vi "Momentum_Killer_V2.vi"(4 "Reverse Power":dbl, 5 "Stop Delay (sec)":dbl=0.5, 6 "Reverse Time (sec)":dbl, 7 "Edge":bool, 9 "Kill Control":bool, 11 "Power Input":dbl) -> (3 "Power Output":dbl)   [LabVIEW 2016]
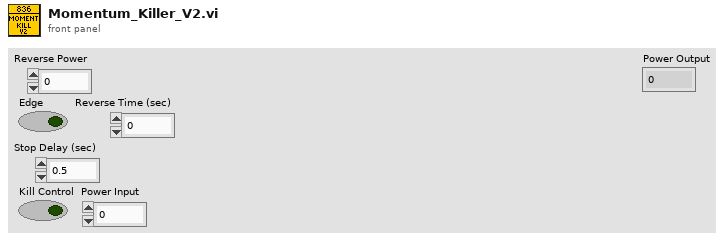
[diagram p1: front panel]
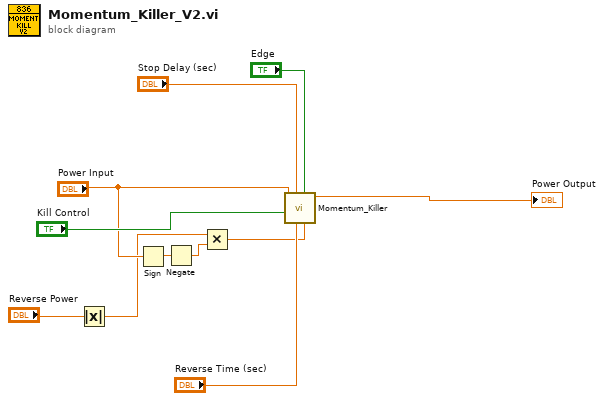
[diagram p0: block diagram]
diagram:
  n1 = Absolute Value(x="Reverse Power") -> (abs(x)=w2:dbl)
  n2 = Sign(1:"Power Input") -> (0:w4:dbl)
  n3 = Negate(x=w4) -> (-x=w5:dbl)
  n4 = Multiply(x=w2, y=w5) -> (x*y=w1:dbl)
  n5 = call <userlib>:"Momentum_Killer.vi"("Reverse Power"=w1, "Edge"="Edge", "Reverse Time (sec)"="Reverse Time (sec)", "Stop Delay (sec)"="Stop Delay (sec)", "Kill Control"="Kill Control", "Power Input"="Power Input") -> ("Power Output"=→"Power Output":dbl)  [unwired: 5 in]
